vi "subGetSourceItemName.vi"(9 "index (1)":u32=1, 11 "Refnum in":refnum<k20>) -> (3 "source name":string)   [LabVIEW 2020, in "SolutionBuilder.lvlib"]
uses:
  SolutionBuilder.lvlib
  <vilib>/xml/NI_XML.lvlib
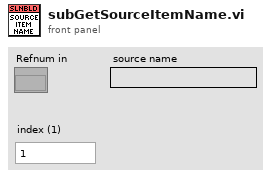
[diagram p1: front panel]
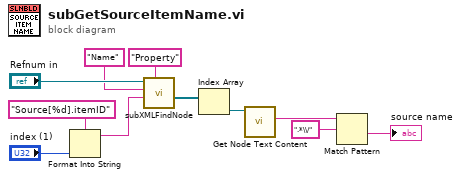
[diagram p0: block diagram]
diagram:
  n1 = Format Into String(format string="Source[%d].itemID" ("Property value"), "index (1)") -> (resulting string=w2:string)  [unwired: 2 in, 1 out]
  n2 = call "subXMLFindNode.vi"("Node name"="Property", "Property value"=w2, "Property name"="Name", "Refnum in"="Refnum in") -> ("Nodes"=w9:refnum<k20>[])  [unwired: 6 in, 1 out]
  n3 = Index Array(array=w9) -> (element=w10:refnum<k20>)  [unwired: 1 in]
  n4 = call <vilib>:"Get Node Text Content.vi"("node in"=w10) -> ("node text"=w6:string)  [unwired: 8 in, 2 out]
  n5 = Match Pattern(string=w6, regular expression=".*\\/") -> (after substring=→"source name":string)  [unwired: 1 in, 3 out]
